vi "LVObject to JSON - Pretty Print - Returns Pretty JSON String.vi"() -> ()   [LabVIEW 2017, in "JSON Serializable Serializer Tests.lvlib"]
uses:
  JSON Serializable Serializer Tests.lvlib
  JSON Serializable Serializer/JSON Serializable Serializer.lvclass
  <vilib>/addons/_JKI Toolkits/Caraya/classes/Assert/Assert Equal Value_Variant.vi
  <vilib>/addons/_JKI Toolkits/Caraya/classes/Test/Test.lvclass
  <vilib>/addons/_JKI Toolkits/Caraya/classes/Assert/Assert.lvclass
  Mock JSON Serializable/Mock JSON Serializable.lvclass
panel:
  out "error out":errorcluster
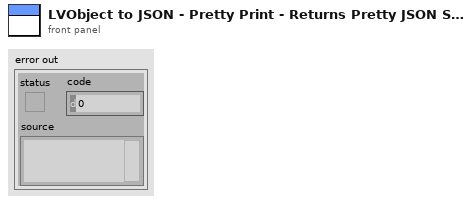
[diagram p1: front panel]
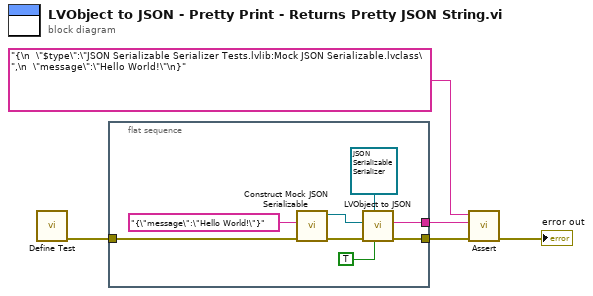
[diagram p0: block diagram]
diagram:
  n1 = call <vilib>:"Define Test.vi"() -> ("error out"=w4:errorcluster)  [unwired: 11 in]
  n2 = flat-sequence {
    tunnel: [w12] -> w5
    tunnel: w4 -> [w10]
    tunnel: [w9] -> w2
    frame #0 {
      n3 = call "Construct Mock JSON Serializable.vi"("error in (no error)"=w10, "To JSON <JSON> (\"{}\")"="{\"message\":\"Hello World!\"}" ("<JSON> (\"{}\")")) -> ("error out"=w8:errorcluster, "Mock JSON Serializable"=w7:refnum<class "Mock JSON Serializable.lvclass">)  [unwired: 8 in]
      n4 = call-dynamic "LVObject to JSON.vi"("Pretty Print?"=TRUE, "JSON Serializable Serializer in"=refnum<class "JSON Serializable Serializer.lvclass"> refnum ("JSON Serializer.lvclass"), "error in (no error)"=w8, "Object"=w7) -> ("error out"=w12:errorcluster, "<JSON>Object"=w9:string)  [unwired: 6 in]
    }
  }
  n5 = call-poly <vilib>:"Assert.vi"("error in (no error)"=w5, "Y"=w2, "X"="{\n  \"$type\":\"JSON Serializable Serializer Tests.lvlib:Mock JSON Serializable.lvclass\",\n  \"message\":\"Hello World!\"\n}") -> ("error out"=→"error out":errorcluster)  [unwired: 8 in]
